vi "Execute.GetRequiredChannels.vi"(8 "error in (no error)":errorcluster, 11 "Path":path=path "C:/Users/blueuser/Desktop/Test.nivsseq") -> (0 "error out":errorcluster, 3 "Channels":string[](array[string]))   [LabVIEW 2013, in "Simple Sequence Editor.lvlib"]
uses:
  Simple Sequence Editor.lvlib
  NationalInstruments.VeriStand.RealTimeSequenceDefinitionApi
  NationalInstruments.VeriStand.DataTypes
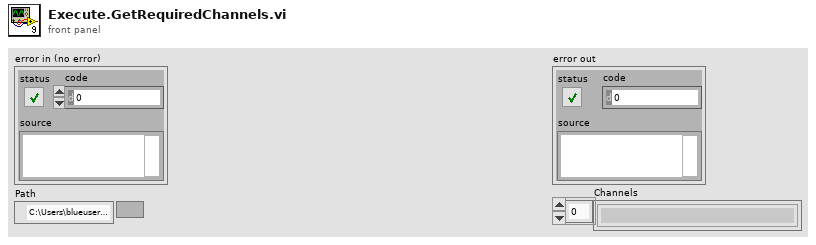
[diagram p1: front panel]
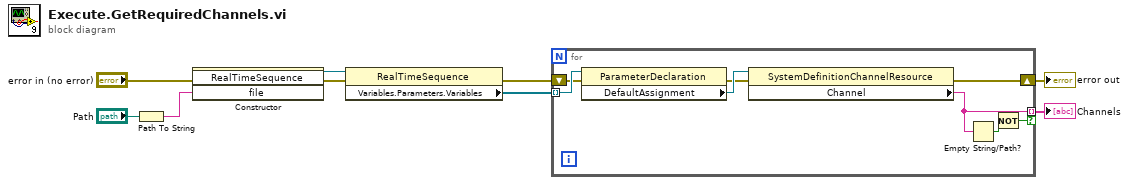
[diagram p0: block diagram]
diagram:
  n1 = Path To String(path="Path") -> (string=w4:string)
  n2 = constructor class="RealTimeSequence"(error in="error in (no error)", "file"=w4) -> (reference out=w9:refnum<k24>, error out=w8:errorcluster)  [unwired: 2 in, 2 out]
  n3 = property class="RealTimeSequence"(reference=w9, error in=w8) -> (error out=w6:errorcluster, "Variables.Parameters.Variables"=w7:refnum<k24>[])  [unwired: 1 out]
  n4 = for {
    tunnel: w7 -> [w17] mode=indexing
    shift-right: [w13] -> w3
    shift-left: w6 -> [w16]
    tunnel: [w12] -> w2 mode=indexing if=w10
    n5 = property class="ParameterDeclaration"(reference=w17, error in=w16) -> (error out=w14:errorcluster, "DefaultAssignment"=w15:refnum<k24>)  [unwired: 1 out]
    n6 = property class="SystemDefinitionChannelResource"(reference=w15, error in=w14) -> (error out=w13:errorcluster, "Channel"=w12:string)  [unwired: 1 out]
    n7 = Empty String/Path?(string/path=w12) -> (empty?=w11:bool)
    n8 = Not(x=w11) -> (.not. x?=w10:bool)
  }
  "error out" <- w3
  "Channels" <- w2
